vi "read_environment.vi"(10 "symbol":string, 11 "Environment in":T3) -> (3 "Expression":T1)   [LabVIEW 2021]
uses:
  Environment.ctl
  Expression.ctl
  ExpressionType.ctl
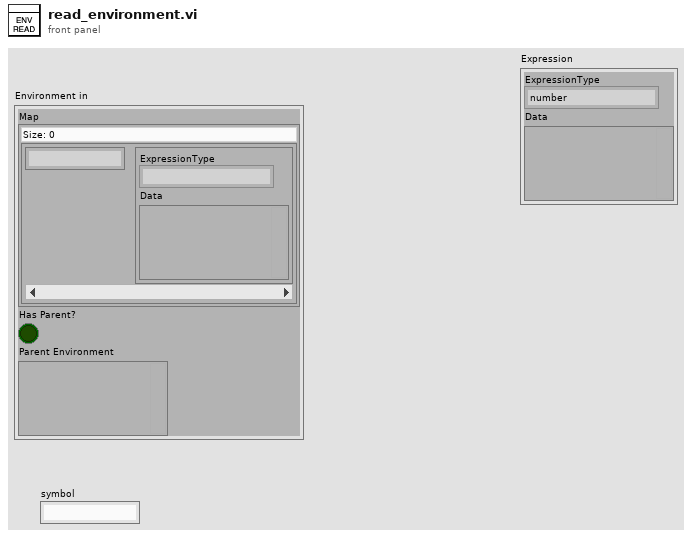
[diagram p1: front panel]
types:
  T1 = typedef "Expression.ctl" = cluster{"ExpressionType":T2, "Data":variant}
  T2 = typedef "ExpressionType.ctl" = enum16{"number", "string", "symbol", "primitive", "list", "closure", "nil", "error"}
  T3 = typedef "Environment.ctl" = cluster{"Map":map{string, T1}, "Has Parent?":bool, "Parent Environment":variant}
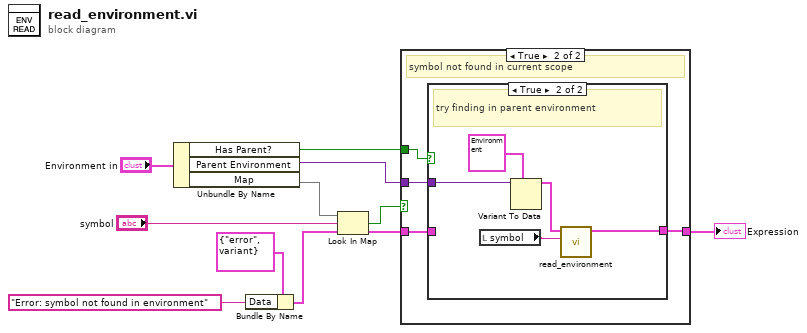
[diagram p0: block diagram]
diagram:
  n1 = Unbundle By Name("Environment in") -> ("Has Parent?"=w2:bool, "Parent Environment"=w1:variant, "Map"=w10:map{string, T1})
  n2 = Bundle By Name(cluster=T1 {"ExpressionType"=enum."error", "Data"=variant} ("Expression"), "Data"="Error: symbol not found in environment") -> (w6:T1)
  n3 = Look In Map(map=w10, key="symbol", default value=w6) -> (key not found?=w5:bool, value=w4:T1)
  n4 = case shown="True" w5 {
    tunnel: w4 -> [w12 w14]
    tunnel: [w12 w15] -> w3
    tunnel: w2 -> [_ w16]
    tunnel: w1 -> [_ w13]
    frame False {
      # "symbol found in current scope, return value"
    }
    frame True {
      # "symbol not found in current scope"
      n5 = case shown="True" w16 {
        tunnel: [w17 w20] -> w15
        tunnel: w14 -> [w17 _]
        tunnel: w13 -> [_ w18]
        frame False {
          # "Uppermost environment; symbol not defined"
        }
        frame True {
          # "try finding in parent environment"
          n6 = local read "symbol"() -> (w21:string)
          n7 = Variant To Data(type=T3 {"Map"={}, "Has Parent?"=FALSE, "Parent Environment"=variant} ("Environment in"), Variant=w18) -> (data=w19:T3)  [unwired: 1 in, 1 out]
          n8 = call "read_environment.vi"("symbol"=w21, "Environment in"=w19) -> ("Expression"=w20:T1)  [unwired: 9 in]
        }
      }
    }
  }
  "Expression" <- w3
